vi "Init.vi"(8 "error in (no error)":errorcluster, 11 "Test Finder in":refnum<class "Test Finder.lvclass">) -> (0 "error out":errorcluster, 3 "Test Finder out":refnum<class "Test Finder.lvclass">)   [LabVIEW 2020, in "Test Finder.lvclass"]
uses:
  Test Finder.lvclass
  Test Finder.lvclass/Test Finder.ctl
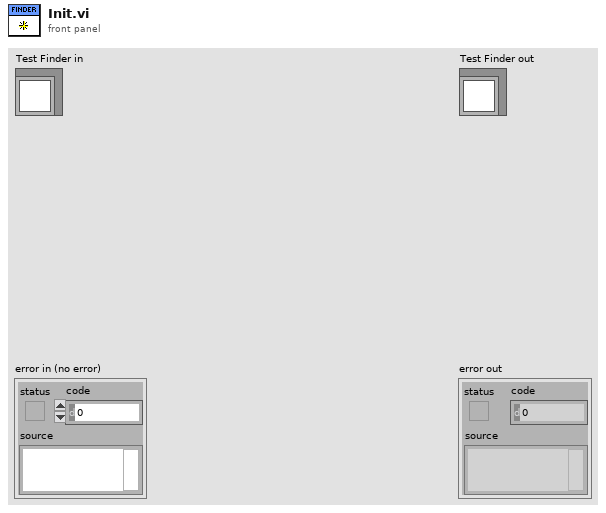
[diagram p1: front panel]
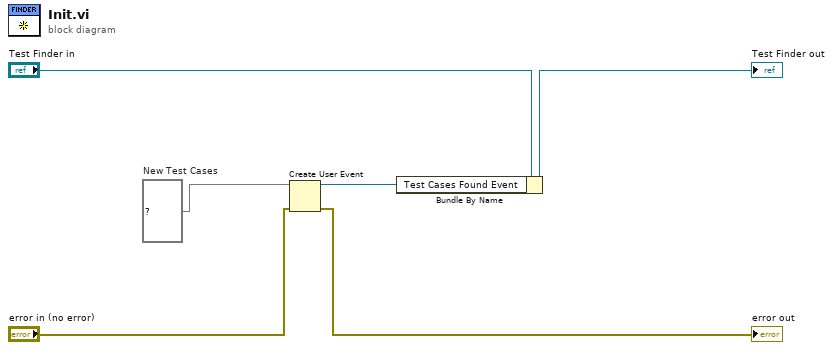
[diagram p0: block diagram]
diagram:
  w1 = set{path} {}  # New Test Cases
  n1 = Create User Event(user event datatype=w1, error in="error in (no error)") -> (user event=w2:refnum<user-event>, error out=→"error out":errorcluster)
  n2 = Bundle By Name(cluster="Test Finder in", "Test Cases Found Event"=w2) -> (→"Test Finder out":refnum<class "Test Finder.lvclass">)
